vi "Get Source Files And Folders.vi"(8 "Error In":errorcluster, 11 "Configuration":T1) -> (0 "Error Out":errorcluster, 1 "All Source Folders":path[](array[path]), 2 "All Source Files":path[](array[path]), 3 "Configuration":T1)   [LabVIEW 2011, in "LVH-Build-Tools.lvlib"]
uses:
  LVH-Build-Tools.lvlib
  Type Defs/Configuration.ctl
  Type Defs/Install Configuration.ctl
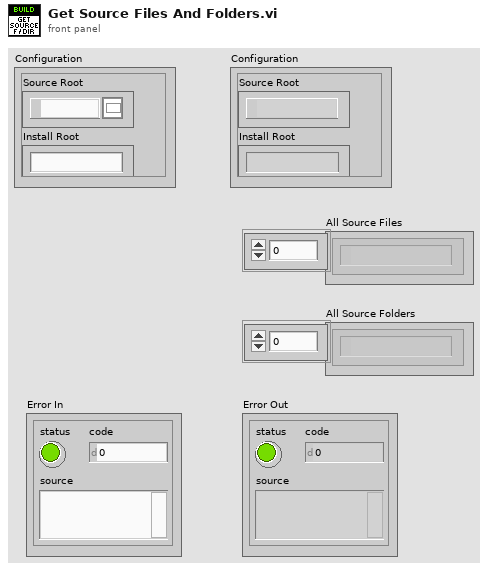
[diagram p1: front panel]
types:
  T1 = typedef "LVH-Build-Tools.lvlib/Configuration.ctl" = cluster{"Source Root":path, "Install Root":string, "Components":string[], "Ignore":string[], "Config Files":path[], "LV Directories":path[], "Install Paths":T2}
  T2 = typedef "LVH-Build-Tools.lvlib/Install Configuration.ctl" = cluster{"LabVIEW Directory":path, "Project Source Config":path}
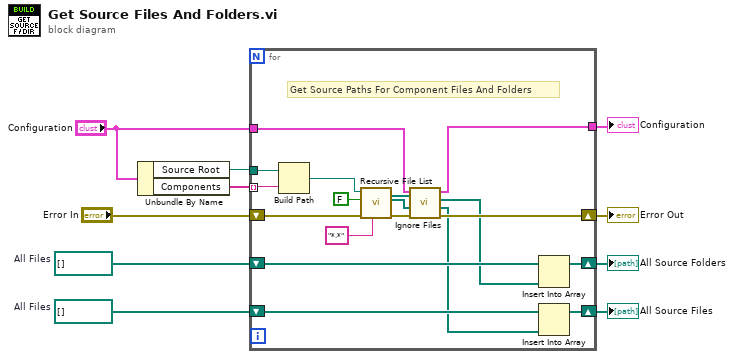
[diagram p0: block diagram]
diagram:
  w7 = path[] []  # All Files
  w6 = path[] []  # All Files
  n1 = Unbundle By Name("Configuration") -> ("Source Root"=w4:path, "Components"=w3:string[])
  n2 = for {
    tunnel: w3 -> [w12] mode=indexing
    tunnel: w4 -> [w13]
    shift-right: [w24] -> w8
    shift-left: w6 -> [w23]
    shift-right: [w21] -> w10
    shift-left: w7 -> [w22]
    shift-right: [w20] -> w9
    shift-left: "Error In" -> [w25]
    tunnel: "Configuration" -> [w17]
    tunnel: [w16] -> w1
    # "Get Source Paths For Component Files And Folders"
    n3 = Build Path(base path=w13, name or relative path=w12) -> (appended path=w11:path)
    n4 = call <vilib>:"Recursive File List.vi"("pattern"="*.*", "error in (no error)"=w25, "Treat LLBs as Folders?"=FALSE, "Folder Path"=w11) -> ("error out"=w28:errorcluster, "All Files in Dir"=w18:path[], "All Folders"=w19:path[])  [unwired: 3 in, 2 out]
    n5 = call "Ignore Files.vi"("Error In"=w28, "All Files"=w18, "All Folders"=w19, "Configuration"=w17) -> ("Error Out"=w20:errorcluster, "All Files"=w14:path[], "All Folders"=w15:path[], "Configuration"=w16:T1)  [unwired: 4 in]
    n6 = Insert Into Array(array=w23, new element=w15) -> (w24:path[])  [unwired: 1 in]
    n7 = Insert Into Array(array=w22, new element=w14) -> (w21:path[])  [unwired: 1 in]
  }
  "All Source Files" <- w10
  "Error Out" <- w9
  "All Source Folders" <- w8
  "Configuration" <- w1
